vi "19572_press_STOP_button.vi"(8 "error in (no error)":errorcluster, 11 "task/channels in":refnum<k21>) -> (0 "error out":errorcluster, 3 "task out":refnum<k21>)   [LabVIEW 2015]
uses:
  <vilib>/DAQmx/write.llb/DAQmx Write (Digital 1D Bool 1Chan 1Samp).vi
  <vilib>/DAQmx/miscellaneous.llb/DAQmx Fill In Error Info.vi
panel:
  # "Press STOP button on CHROMA 19572"
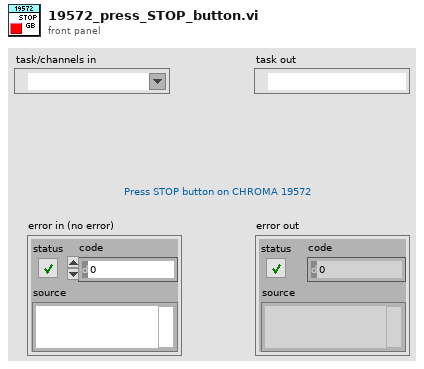
[diagram p1: front panel]
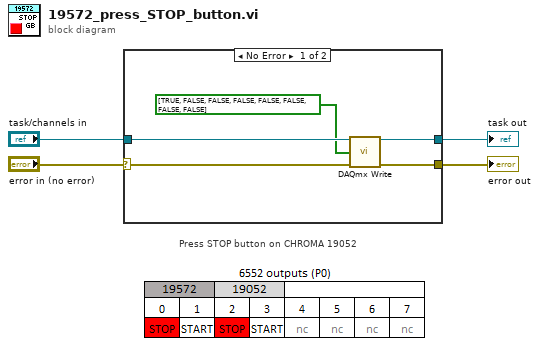
[diagram p0: block diagram]
diagram:
  # "Press STOP button on CHROMA 19052"
  n1 = case shown="No Error" "error in (no error)" {
    selector: "error in (no error)" -> [w8 w10]
    tunnel: "task/channels in" -> [w9 w11]
    tunnel: [w5 w10] -> w2
    tunnel: [w6 w11] -> w1
    frame No Error {
      n2 = call-poly <vilib>:"DAQmx Write.vi"("task/channels in"=w9, "data"=bool[] [TRUE, FALSE, FALSE, FALSE, FALSE, FALSE, FALSE, FALSE], "error in"=w8) -> ("task out"=w6:refnum<k21>, "error out"=w5:errorcluster)  [unwired: 10 in, 1 out]
    }
    frame Error {
    }
  }
  "error out" <- w2
  "task out" <- w1
